vi "20Data.vi"(8 "error in":errorcluster, 11 "VISA resource name":refnum<visa-resource-name>) -> (0 "error out":errorcluster, 1 "Mean Z":dbl format="%0.2f", 2 "Mean Y":dbl format="%0.2f", 3 "VISA Refnum  out":refnum<visa-resource-name>)   [LabVIEW 2020]
uses:
  <vilib>/Analysis/baseanly.llb/Mean (DBL).vi
  <vilib>/Analysis/NI_AALBase.lvlib
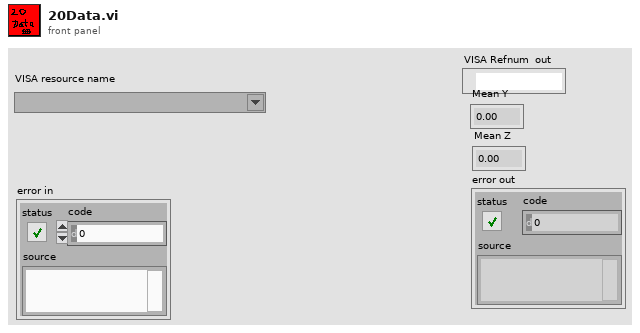
[diagram p1: front panel]
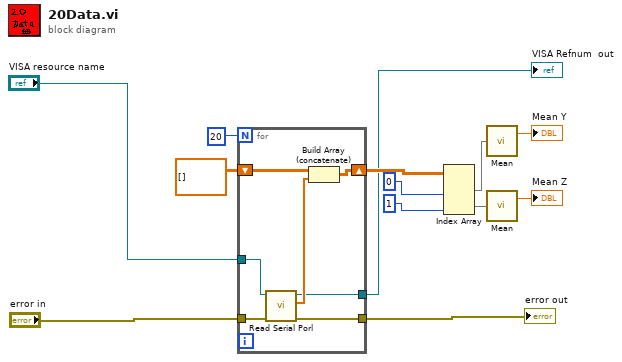
[diagram p0: block diagram]
diagram:
  n1 = for {
    N: 20 -> [_]
    tunnel: "VISA resource name" -> [w20]
    shift-right: [w18] -> w4
    shift-left: dbl[][] [] -> [w19]
    tunnel: [w17] -> w5
    tunnel: "error in" -> [w16]
    tunnel: [w14] -> w3
    n2 = call "Read Serial Porl.vi"("error in (no error)"=w16, "VISA Refnum in"=w20) -> ("error out"=w17:errorcluster, "Array"=w15:dbl[], "VISA Refnum  out"=w14:refnum<visa-resource-name>)  [unwired: 6 in, 1 out]
    n3 = Build Array (concatenate)(w19, w15) -> (w18:dbl[][])
  }
  "error out" <- w5
  "VISA Refnum  out" <- w3
  n4 = Index Array(array=w4, index (col) #1=0 ("disabled index (col)"), index (col) #2=1 ("index (col)")) -> (element #1=w11:dbl[], element #2=w10:dbl[])  [unwired: 2 in]
  n5 = call-poly <vilib>:"Mean.vi"("X"=w11) -> ("mean"=→"Mean Y":dbl)  [unwired: 1 out]
  n6 = call-poly <vilib>:"Mean.vi"("X"=w10) -> ("mean"=→"Mean Z":dbl)  [unwired: 1 out]
